vi "Resolve Group State.vi"(4 "Logger States":T1[](array[typedef])) -> (7 "Group State":T1)   [LabVIEW 2020, in "VolatusData.lvlib" / "Log Manager Module.lvclass"]
uses:
  Log Manager Module.lvclass
  Logger State.ctl
  Log Manager Module.lvclass/Log Manager Module.ctl
  VolatusData.lvlib
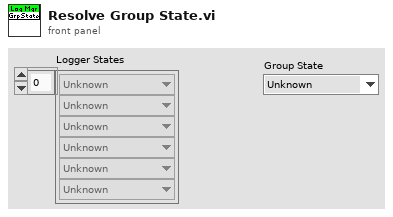
[diagram p1: front panel]
types:
  T1 = typedef "VolatusData.lvlib/Logger State.ctl" = enum16{"Unknown", "Idle", "Preparing", "Ready", "Logging", "Stopping"}
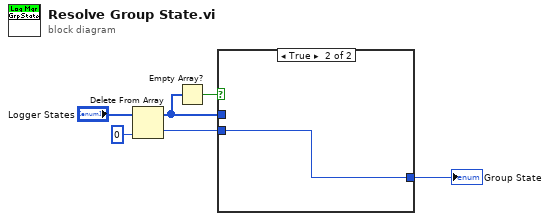
[diagram p0: block diagram]
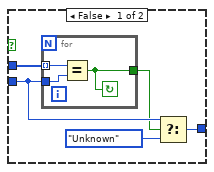
[diagram p2: hidden frame]
diagram:
  n1 = Delete From Array(array="Logger States", index=0) -> (deleted portion=w4:T1, array with subset deleted=w2:T1[])  [unwired: 1 in]
  n2 = Empty Array?(array=w2) -> (empty?=w1:bool)
  n3 = case shown="True" w1 {
    tunnel: w4 -> [w11 w15]
    tunnel: [w8 w15] -> w3
    tunnel: w2 -> [w7 _]
    frame False {
      n4 = for {
        tunnel: w7 -> [w14] mode=indexing
        tunnel: w11 -> [w13]
        tunnel: [w12] -> w10
        stop <- w12 continue-if-true
        n5 = Equal?(x=w14, y=w13) -> (x = y?=w12:bool)
      }
      n6 = Select(t=w11, s=w10, f=Logger_State."Unknown") -> (s? t:f=w8:T1)
    }
    frame True {
    }
  }
  "Group State" <- w3
